vi "zadanie_1_sortowanie.vi"() -> ()   [LabVIEW 2024]
panel:
  in  "Input Array":dbl[][](array[numeric])
  in  "Select row":dbl
  in  "Select column":dbl
  in  "Column/Row":bool
  out "Output Array":dbl[][](array[numeric])
  in  "stop":bool
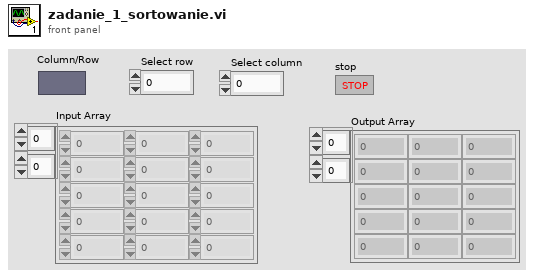
[diagram p1: front panel]
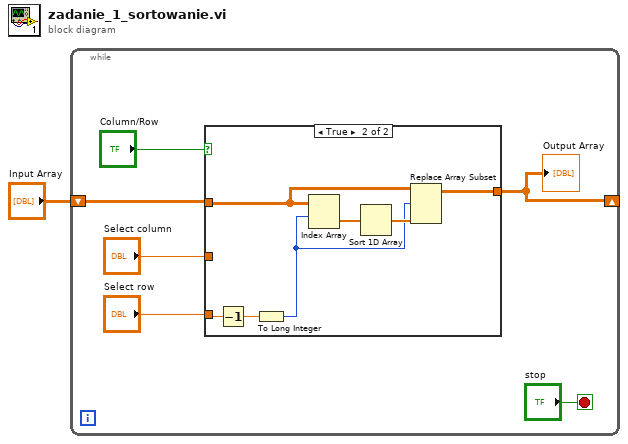
[diagram p0: block diagram]
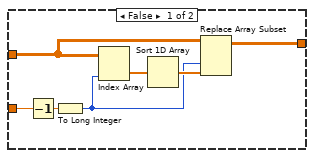
[diagram p2: hidden frame]
diagram:
  n1 = while {
    shift-right: [w2] -> _
    shift-left: "Input Array" -> [w3]
    stop <- "stop" stop-if-true
    n2 = case shown="True" "Column/Row" {
      tunnel: "Select column" -> [w10 _]
      tunnel: "Select row" -> [_ w21]
      tunnel: w3 -> [w12 w20]
      tunnel: [w11 w16] -> w2
      frame False {
        n3 = Decrement(x=w10) -> (x-1=w9:dbl)
        n4 = To Long Integer(number=w9) -> (32bit integer=w8:i32)
        n5 = Index Array(array=w12, index (col)=w8) -> (element=w14:dbl[])  [unwired: 1 in]
        n6 = Sort 1D Array(array=w14) -> (sorted array=w13:dbl[])
        n7 = Replace Array Subset(array=w12, new element=w13, index (col)=w8) -> (w11:dbl[][])  [unwired: 1 in]
      }
      frame True {
        n8 = Decrement(x=w21) -> (x-1=w19:dbl)
        n9 = To Long Integer(number=w19) -> (32bit integer=w15:i32)
        n10 = Index Array(array=w20, index (row)=w15) -> (element=w18:dbl[])  [unwired: 1 in]
        n11 = Sort 1D Array(array=w18) -> (sorted array=w17:dbl[])
        n12 = Replace Array Subset(array=w20, new element=w17, index (row)=w15) -> (w16:dbl[][])  [unwired: 1 in]
      }
    }
    "Output Array" <- w2
  }
